vi "Write RF Waveform Database.vi"(8 "error in (no error)":errorcluster, 10 "WFM MNGR":refnum<class "QPA MSMT Waveform Manager.lvclass">, 11 "QPA Measurement in":refnum<class "QPA Measurement.lvclass">=refnum) -> (0 "error out":errorcluster, 3 "QPA Measurement out":refnum<class "QPA Measurement.lvclass">)   [LabVIEW 2016, in "QPA Measurement.lvlib" / "QPA Measurement.lvclass"]
uses:
  QPA Measurement.lvclass
  Waveform Manager/QPA MSMT Waveform Manager.lvclass
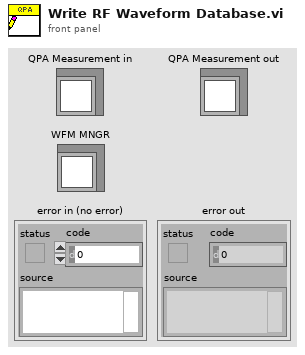
[diagram p1: front panel]
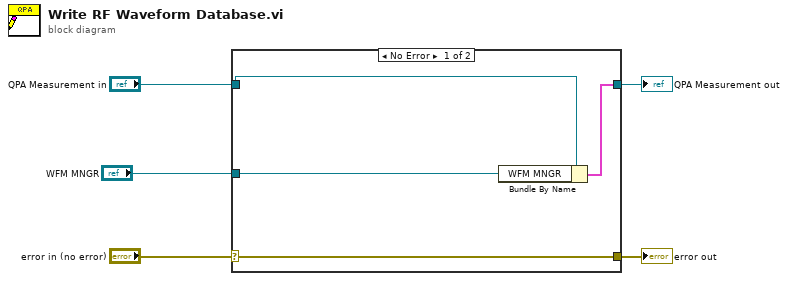
[diagram p0: block diagram]
diagram:
  n1 = case shown="No Error" "error in (no error)" {
    selector: "error in (no error)" -> [w9 w10]
    tunnel: [w9 w10] -> w4
    tunnel: [w7 w11] -> w2
    tunnel: "QPA Measurement in" -> [w8 w11]
    tunnel: "WFM MNGR" -> [w6 _]
    frame No Error {
      n2 = Bundle By Name(cluster=w8, "WFM MNGR"=w6) -> (w7:cluster{})
    }
    frame Error {
    }
  }
  "error out" <- w4
  "QPA Measurement out" <- w2
